vi "create cancellation token.vi"(8 "error in":errorcluster) -> (0 "error out":errorcluster, 3 "cancel token out":refnum<class "cancel token.lvclass">)   [LabVIEW 2013, in "cancel token.lvclass"]
uses:
  cancel token.lvclass
  cancel token.lvclass/cancel token.ctl
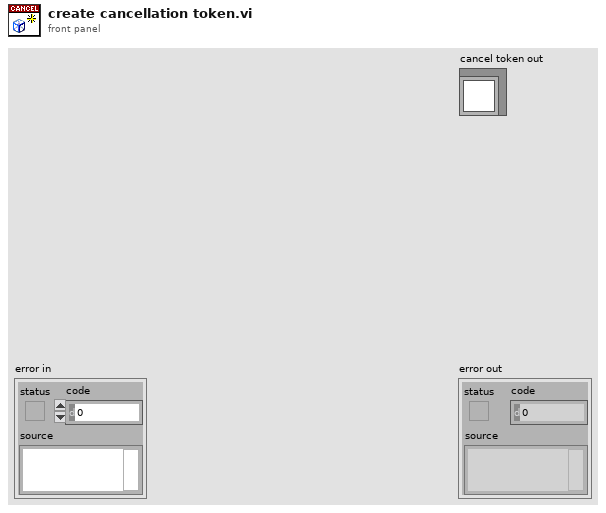
[diagram p1: front panel]
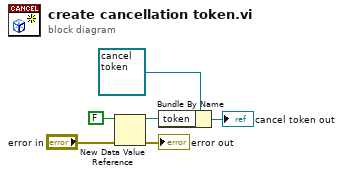
[diagram p0: block diagram]
diagram:
  n1 = New Data Value Reference(data value=FALSE, error in="error in") -> (data value reference=w1:refnum<data-value>, error out=→"error out":errorcluster)
  n2 = Bundle By Name(cluster=refnum<class "cancel token.lvclass"> refnum ("cancel token in"), "token"=w1) -> (→"cancel token out":refnum<class "cancel token.lvclass">)
